vi "chamber control mockup.vi"() -> ()   [LabVIEW 2013]
uses:
  dconners svn copy/TemperatureLogger/controls/TabControl.ctl
  dconners svn copy/TemperatureLogger/controls/TemperatureControlCluster2.ctl
  dconners svn copy/TemperatureLogger/controls/outputcluster.ctl
panel:
  in  "Save freq (seconds between samples)":dbl
  in  "Log note":bool
  in  "Notes":string
  out "Chiller alarm":bool
  out "Free GB":dbl
  in  "Data storage location":path
  in  "Chiller flow speed":u16(ring) items=["Low", "Medium", "High"]
  in  "Chiller process value":dbl
  in  "Chiller setpoint":dbl
  out "Profile running":bool
  in  "Big Chamber setpoint 3":dbl
  out "Big Chamber process value 3":dbl
  in  "Little Chamber setpoint 3":dbl
  out "Little Chamber process value 3":dbl
  in  "Big Chamber setpoint 2":dbl
  out "Big Chamber process value 2":dbl
  in  "Little Chamber setpoint 2":dbl
  out "Little Chamber process value 2":dbl
  in  "Relay 3":bool
  in  "Relay 2":bool
  in  "Relay 4":bool
  in  "Relay 1":bool
  in  "Tab Control":T1(tab)
  in  "Popout to new window 6":bool
  in  "Tab Control 7":T2
  in  "String 18":string
  in  "String 17":string
  in  "String 16":string
  in  "String 15":string
  in  "String 14":string
  in  "String 13":string
  in  "String 12":string
  in  "String 11":string
  in  "String 10":string
  in  "String 9":string
  in  "String 8":string
  in  "String 7":string
  in  "String 6":string
  in  "String 5":string
  in  "String 4":string
  in  "String 3":string
  in  "String 2":string
  out "DisplayCluster 6":T3={"Thermometer 2"=0.0, "Temperature Chart 4"=[{"t0"=timestamp(3419368924.4957023 s since 1904-01-01), "dt"=1.0, "Y"=[23.012484100583272], "attributes"=variant("NI_ChannelName"=variant(string "ai0"), "NI_UnitDescription"=variant(string "Deg C"))}, {"t0"=timestamp(3419368924.4957023 s since 1904-01-01), "dt"=1.0, "Y"=[23.20749068697193], "attributes"=variant("NI_ChannelName"=variant(string "ai1"), "NI_UnitDescription"=variant(string "Deg C"))}, {"t0"=timestamp(3419368924.4957023 s since 1904-01-01), "dt"=1.0, "Y"=[23.4994745351067], "attributes"=variant("NI_ChannelName"=variant(string "ai2"), "NI_UnitDescription"=variant(string "Deg C"))}], "Alarm"=FALSE, "Thermometer"=0.0, "File Path"=""} {"Thermometer" scale=0.0..100.0; "Thermometer 2" scale=0.0..100.0}
  out "Temperatures 6":dbl[](array[numeric]) format="%#.2f"
  in  "Save Data 6":bool=TRUE
  in  "Log File Path 6":path=path "c:/Temp/Data"
  out "DAQmx Device Name 6":tag="cDAQ2Mod1"
  out "Errors 6":errorcluster
  in  "Number of channels 6":i32=1 min=1 max=16 step=1
  in  "sample/S 6":dbl=1.0 min=0.1 max=75.0 step=0.1
  in  "Alarm recipients 6":string[](array[string])=["dconnors@intven.com"]
  in  "Upper Alarm 6":dbl=150.0
  in  "Lower Alarm 6":dbl=-150.0
  in  "Email Enable 6":bool
  in  "Cluster 7":T4={"Channel Setup"=[{"Channel #"=1, "TC TYPE"=10086, "Name"=""}, {"Channel #"=5, "TC TYPE"=10086, "Name"=""}, {"Channel #"=9, "TC TYPE"=10086, "Name"=""}, {"Channel #"=13, "TC TYPE"=10086, "Name"=""}], "Channel Setup 2"=[{"Channel #"=1, "TC TYPE"=10086, "Name"=""}, {"Channel #"=5, "TC TYPE"=10086, "Name"=""}, {"Channel #"=9, "TC TYPE"=10086, "Name"=""}, {"Channel #"=13, "TC TYPE"=10086, "Name"=""}], "Channel Setup 3"=[{"Channel #"=1, "TC TYPE"=10086, "Name"=""}, {"Channel #"=5, "TC TYPE"=10086, "Name"=""}, {"Channel #"=9, "TC TYPE"=10086, "Name"=""}, {"Channel #"=13, "TC TYPE"=10086, "Name"=""}], "Channel Setup 4"=[{"Channel #"=1, "TC TYPE"=10086, "Name"=""}, {"Channel #"=5, "TC TYPE"=10086, "Name"=""}, {"Channel #"=9, "TC TYPE"=10086, "Name"=""}, {"Channel #"=13, "TC TYPE"=10086, "Name"=""}]} {"Channel Setup 4"."TC TYPE" items=["J"=10072, "K"=10073, "N"=10077, "R"=10082, "S"=10085, "T"=10086, "B"=10047, "E"=10055]; "Channel Setup 4"."Channel #" min=1 max=16 step=1; "Channel Setup 3"."TC TYPE" items=["J"=10072, "K"=10073, "N"=10077, "R"=10082, "S"=10085, "T"=10086, "B"=10047, "E"=10055]; "Channel Setup 3"."Channel #" min=1 max=16 step=1; "Channel Setup 2"."TC TYPE" items=["J"=10072, "K"=10073, "N"=10077, "R"=10082, "S"=10085, "T"=10086, "B"=10047, "E"=10055]; "Channel Setup 2"."Channel #" min=1 max=16 step=1; "Channel Setup"."TC TYPE" items=["J"=10072, "K"=10073, "N"=10077, "R"=10082, "S"=10085, "T"=10086, "B"=10047, "E"=10055]; "Channel Setup"."Channel #" min=1 max=16 step=1}
  out "IP Address 6":string=" "
  in  "Minutes between emails 6":dbl=10.0
  in  "Popout to new window":bool
  in  "Tab Control 2":T2
  in  "String":string
  out "DisplayCluster":T3={"Thermometer 2"=0.0, "Temperature Chart 4"=[{"t0"=timestamp(3419368924.4957023 s since 1904-01-01), "dt"=1.0, "Y"=[23.012484100583272], "attributes"=variant("NI_ChannelName"=variant(string "ai0"), "NI_UnitDescription"=variant(string "Deg C"))}, {"t0"=timestamp(3419368924.4957023 s since 1904-01-01), "dt"=1.0, "Y"=[23.20749068697193], "attributes"=variant("NI_ChannelName"=variant(string "ai1"), "NI_UnitDescription"=variant(string "Deg C"))}, {"t0"=timestamp(3419368924.4957023 s since 1904-01-01), "dt"=1.0, "Y"=[23.4994745351067], "attributes"=variant("NI_ChannelName"=variant(string "ai2"), "NI_UnitDescription"=variant(string "Deg C"))}], "Alarm"=FALSE, "Thermometer"=0.0, "File Path"=""} {"Thermometer" scale=0.0..100.0; "Thermometer 2" scale=0.0..100.0}
  out "Temperatures":dbl[](array[numeric]) format="%#.2f"
  in  "Reset max/min":bool
  in  "Save Data":bool=TRUE
  in  "Log File Path":path=path "c:/Temp/Data"
  out "DAQmx Device Name":tag="cDAQ2Mod1"
  out "Errors":errorcluster
  in  "Number of channels":i32=1 min=1 max=16 step=1
  in  "sample/S":dbl=1.0 min=0.1 max=75.0 step=0.1
  in  "Alarm recipients":string[](array[string])=["dconnors@intven.com"]
  in  "Upper Alarm":dbl=150.0
  in  "Lower Alarm":dbl=-150.0
  in  "Email Enable":bool
  in  "Cluster 2":T4={"Channel Setup"=[{"Channel #"=1, "TC TYPE"=10086, "Name"=""}, {"Channel #"=5, "TC TYPE"=10086, "Name"=""}, {"Channel #"=9, "TC TYPE"=10086, "Name"=""}, {"Channel #"=13, "TC TYPE"=10086, "Name"=""}], "Channel Setup 2"=[{"Channel #"=1, "TC TYPE"=10086, "Name"=""}, {"Channel #"=5, "TC TYPE"=10086, "Name"=""}, {"Channel #"=9, "TC TYPE"=10086, "Name"=""}, {"Channel #"=13, "TC TYPE"=10086, "Name"=""}], "Channel Setup 3"=[{"Channel #"=1, "TC TYPE"=10086, "Name"=""}, {"Channel #"=5, "TC TYPE"=10086, "Name"=""}, {"Channel #"=9, "TC TYPE"=10086, "Name"=""}, {"Channel #"=13, "TC TYPE"=10086, "Name"=""}], "Channel Setup 4"=[{"Channel #"=1, "TC TYPE"=10086, "Name"=""}, {"Channel #"=5, "TC TYPE"=10086, "Name"=""}, {"Channel #"=9, "TC TYPE"=10086, "Name"=""}, {"Channel #"=13, "TC TYPE"=10086, "Name"=""}]} {"Channel Setup 4"."TC TYPE" items=["J"=10072, "K"=10073, "N"=10077, "R"=10082, "S"=10085, "T"=10086, "B"=10047, "E"=10055]; "Channel Setup 4"."Channel #" min=1 max=16 step=1; "Channel Setup 3"."TC TYPE" items=["J"=10072, "K"=10073, "N"=10077, "R"=10082, "S"=10085, "T"=10086, "B"=10047, "E"=10055]; "Channel Setup 3"."Channel #" min=1 max=16 step=1; "Channel Setup 2"."TC TYPE" items=["J"=10072, "K"=10073, "N"=10077, "R"=10082, "S"=10085, "T"=10086, "B"=10047, "E"=10055]; "Channel Setup 2"."Channel #" min=1 max=16 step=1; "Channel Setup"."TC TYPE" items=["J"=10072, "K"=10073, "N"=10077, "R"=10082, "S"=10085, "T"=10086, "B"=10047, "E"=10055]; "Channel Setup"."Channel #" min=1 max=16 step=1}
  out "IP Address":string=" "
  in  "Minutes between emails":dbl=10.0
  in  "Popout to new window 7":bool
  in  "Tab Control 8":T2
  in  "String 36":string
  in  "String 35":string
  in  "String 34":string
  in  "String 33":string
  in  "String 32":string
  in  "String 31":string
  in  "String 30":string
  in  "String 29":string
  in  "String 28":string
  in  "String 27":string
  in  "String 26":string
  in  "String 25":string
  in  "String 24":string
  in  "String 23":string
  in  "String 22":string
  in  "String 21":string
  in  "String 20":string
  out "DisplayCluster 7":T3={"Thermometer 2"=0.0, "Temperature Chart 4"=[{"t0"=timestamp(3419368924.4957023 s since 1904-01-01), "dt"=1.0, "Y"=[23.012484100583272], "attributes"=variant("NI_ChannelName"=variant(string "ai0"), "NI_UnitDescription"=variant(string "Deg C"))}, {"t0"=timestamp(3419368924.4957023 s since 1904-01-01), "dt"=1.0, "Y"=[23.20749068697193], "attributes"=variant("NI_ChannelName"=variant(string "ai1"), "NI_UnitDescription"=variant(string "Deg C"))}, {"t0"=timestamp(3419368924.4957023 s since 1904-01-01), "dt"=1.0, "Y"=[23.4994745351067], "attributes"=variant("NI_ChannelName"=variant(string "ai2"), "NI_UnitDescription"=variant(string "Deg C"))}], "Alarm"=FALSE, "Thermometer"=0.0, "File Path"=""} {"Thermometer" scale=0.0..100.0; "Thermometer 2" scale=0.0..100.0}
  out "Temperatures 7":dbl[](array[numeric]) format="%#.2f"
  in  "Save Data 7":bool=TRUE
  in  "Log File Path 7":path=path "c:/Temp/Data"
  out "DAQmx Device Name 7":tag="cDAQ2Mod1"
  out "Errors 7":errorcluster
  in  "Number of channels 7":i32=1 min=1 max=16 step=1
  in  "sample/S 7":dbl=1.0 min=0.1 max=75.0 step=0.1
  in  "Alarm recipients 7":string[](array[string])=["dconnors@intven.com"]
  in  "Upper Alarm 7":dbl=150.0
  in  "Lower Alarm 7":dbl=-150.0
  in  "Email Enable 7":bool
  in  "Cluster 8":T4={"Channel Setup"=[{"Channel #"=1, "TC TYPE"=10086, "Name"=""}, {"Channel #"=5, "TC TYPE"=10086, "Name"=""}, {"Channel #"=9, "TC TYPE"=10086, "Name"=""}, {"Channel #"=13, "TC TYPE"=10086, "Name"=""}], "Channel Setup 2"=[{"Channel #"=1, "TC TYPE"=10086, "Name"=""}, {"Channel #"=5, "TC TYPE"=10086, "Name"=""}, {"Channel #"=9, "TC TYPE"=10086, "Name"=""}, {"Channel #"=13, "TC TYPE"=10086, "Name"=""}], "Channel Setup 3"=[{"Channel #"=1, "TC TYPE"=10086, "Name"=""}, {"Channel #"=5, "TC TYPE"=10086, "Name"=""}, {"Channel #"=9, "TC TYPE"=10086, "Name"=""}, {"Channel #"=13, "TC TYPE"=10086, "Name"=""}], "Channel Setup 4"=[{"Channel #"=1, "TC TYPE"=10086, "Name"=""}, {"Channel #"=5, "TC TYPE"=10086, "Name"=""}, {"Channel #"=9, "TC TYPE"=10086, "Name"=""}, {"Channel #"=13, "TC TYPE"=10086, "Name"=""}]} {"Channel Setup 4"."TC TYPE" items=["J"=10072, "K"=10073, "N"=10077, "R"=10082, "S"=10085, "T"=10086, "B"=10047, "E"=10055]; "Channel Setup 4"."Channel #" min=1 max=16 step=1; "Channel Setup 3"."TC TYPE" items=["J"=10072, "K"=10073, "N"=10077, "R"=10082, "S"=10085, "T"=10086, "B"=10047, "E"=10055]; "Channel Setup 3"."Channel #" min=1 max=16 step=1; "Channel Setup 2"."TC TYPE" items=["J"=10072, "K"=10073, "N"=10077, "R"=10082, "S"=10085, "T"=10086, "B"=10047, "E"=10055]; "Channel Setup 2"."Channel #" min=1 max=16 step=1; "Channel Setup"."TC TYPE" items=["J"=10072, "K"=10073, "N"=10077, "R"=10082, "S"=10085, "T"=10086, "B"=10047, "E"=10055]; "Channel Setup"."Channel #" min=1 max=16 step=1}
  out "IP Address 7":string=" "
  in  "Minutes between emails 7":dbl=10.0
  in  "Popout to new window 2":bool
  in  "Tab Control 3":T2
  in  "String 19":string
  out "DisplayCluster 2":T3={"Thermometer 2"=0.0, "Temperature Chart 4"=[{"t0"=timestamp(3419368924.4957023 s since 1904-01-01), "dt"=1.0, "Y"=[23.012484100583272], "attributes"=variant("NI_ChannelName"=variant(string "ai0"), "NI_UnitDescription"=variant(string "Deg C"))}, {"t0"=timestamp(3419368924.4957023 s since 1904-01-01), "dt"=1.0, "Y"=[23.20749068697193], "attributes"=variant("NI_ChannelName"=variant(string "ai1"), "NI_UnitDescription"=variant(string "Deg C"))}, {"t0"=timestamp(3419368924.4957023 s since 1904-01-01), "dt"=1.0, "Y"=[23.4994745351067], "attributes"=variant("NI_ChannelName"=variant(string "ai2"), "NI_UnitDescription"=variant(string "Deg C"))}], "Alarm"=FALSE, "Thermometer"=0.0, "File Path"=""} {"Thermometer" scale=0.0..100.0; "Thermometer 2" scale=0.0..100.0}
  out "Temperatures 2":dbl[](array[numeric]) format="%#.2f"
  in  "Reset max/min 2":bool
  in  "Save Data 2":bool=TRUE
  in  "Log File Path 2":path=path "c:/Temp/Data"
  out "DAQmx Device Name 2":tag="cDAQ2Mod1"
  out "Errors 2":errorcluster
  in  "Number of channels 2":i32=1 min=1 max=16 step=1
  in  "sample/S 2":dbl=1.0 min=0.1 max=75.0 step=0.1
  in  "Alarm recipients 2":string[](array[string])=["dconnors@intven.com"]
  in  "Upper Alarm 2":dbl=150.0
  in  "Lower Alarm 2":dbl=-150.0
  in  "Email Enable 2":bool
  in  "Cluster 3":T4={"Channel Setup"=[{"Channel #"=1, "TC TYPE"=10086, "Name"=""}, {"Channel #"=5, "TC TYPE"=10086, "Name"=""}, {"Channel #"=9, "TC TYPE"=10086, "Name"=""}, {"Channel #"=13, "TC TYPE"=10086, "Name"=""}], "Channel Setup 2"=[{"Channel #"=1, "TC TYPE"=10086, "Name"=""}, {"Channel #"=5, "TC TYPE"=10086, "Name"=""}, {"Channel #"=9, "TC TYPE"=10086, "Name"=""}, {"Channel #"=13, "TC TYPE"=10086, "Name"=""}], "Channel Setup 3"=[{"Channel #"=1, "TC TYPE"=10086, "Name"=""}, {"Channel #"=5, "TC TYPE"=10086, "Name"=""}, {"Channel #"=9, "TC TYPE"=10086, "Name"=""}, {"Channel #"=13, "TC TYPE"=10086, "Name"=""}], "Channel Setup 4"=[{"Channel #"=1, "TC TYPE"=10086, "Name"=""}, {"Channel #"=5, "TC TYPE"=10086, "Name"=""}, {"Channel #"=9, "TC TYPE"=10086, "Name"=""}, {"Channel #"=13, "TC TYPE"=10086, "Name"=""}]} {"Channel Setup 4"."TC TYPE" items=["J"=10072, "K"=10073, "N"=10077, "R"=10082, "S"=10085, "T"=10086, "B"=10047, "E"=10055]; "Channel Setup 4"."Channel #" min=1 max=16 step=1; "Channel Setup 3"."TC TYPE" items=["J"=10072, "K"=10073, "N"=10077, "R"=10082, "S"=10085, "T"=10086, "B"=10047, "E"=10055]; "Channel Setup 3"."Channel #" min=1 max=16 step=1; "Channel Setup 2"."TC TYPE" items=["J"=10072, "K"=10073, "N"=10077, "R"=10082, "S"=10085, "T"=10086, "B"=10047, "E"=10055]; "Channel Setup 2"."Channel #" min=1 max=16 step=1; "Channel Setup"."TC TYPE" items=["J"=10072, "K"=10073, "N"=10077, "R"=10082, "S"=10085, "T"=10086, "B"=10047, "E"=10055]; "Channel Setup"."Channel #" min=1 max=16 step=1}
  out "IP Address 2":string=" "
  in  "Minutes between emails 2":dbl=10.0
  in  "Popout to new window 8":bool
  in  "Tab Control 9":T2
  in  "String 54":string
  in  "String 53":string
  in  "String 52":string
  in  "String 51":string
  in  "String 50":string
  in  "String 49":string
  in  "String 48":string
  in  "String 47":string
  in  "String 46":string
  in  "String 45":string
  in  "String 44":string
  in  "String 43":string
  in  "String 42":string
  in  "String 41":string
  in  "String 40":string
  in  "String 39":string
  in  "String 38":string
  out "DisplayCluster 8":T3={"Thermometer 2"=0.0, "Temperature Chart 4"=[{"t0"=timestamp(3419368924.4957023 s since 1904-01-01), "dt"=1.0, "Y"=[23.012484100583272], "attributes"=variant("NI_ChannelName"=variant(string "ai0"), "NI_UnitDescription"=variant(string "Deg C"))}, {"t0"=timestamp(3419368924.4957023 s since 1904-01-01), "dt"=1.0, "Y"=[23.20749068697193], "attributes"=variant("NI_ChannelName"=variant(string "ai1"), "NI_UnitDescription"=variant(string "Deg C"))}, {"t0"=timestamp(3419368924.4957023 s since 1904-01-01), "dt"=1.0, "Y"=[23.4994745351067], "attributes"=variant("NI_ChannelName"=variant(string "ai2"), "NI_UnitDescription"=variant(string "Deg C"))}], "Alarm"=FALSE, "Thermometer"=0.0, "File Path"=""} {"Thermometer" scale=0.0..100.0; "Thermometer 2" scale=0.0..100.0}
  out "Temperatures 8":dbl[](array[numeric]) format="%#.2f"
  in  "Save Data 8":bool=TRUE
  in  "Log File Path 8":path=path "c:/Temp/Data"
  out "DAQmx Device Name 8":tag="cDAQ2Mod1"
  out "Errors 8":errorcluster
  in  "Number of channels 8":i32=1 min=1 max=16 step=1
  in  "sample/S 8":dbl=1.0 min=0.1 max=75.0 step=0.1
  in  "Alarm recipients 8":string[](array[string])=["dconnors@intven.com"]
  in  "Upper Alarm 8":dbl=150.0
  in  "Lower Alarm 8":dbl=-150.0
  in  "Email Enable 8":bool
  in  "Cluster 9":T4={"Channel Setup"=[{"Channel #"=1, "TC TYPE"=10086, "Name"=""}, {"Channel #"=5, "TC TYPE"=10086, "Name"=""}, {"Channel #"=9, "TC TYPE"=10086, "Name"=""}, {"Channel #"=13, "TC TYPE"=10086, "Name"=""}], "Channel Setup 2"=[{"Channel #"=1, "TC TYPE"=10086, "Name"=""}, {"Channel #"=5, "TC TYPE"=10086, "Name"=""}, {"Channel #"=9, "TC TYPE"=10086, "Name"=""}, {"Channel #"=13, "TC TYPE"=10086, "Name"=""}], "Channel Setup 3"=[{"Channel #"=1, "TC TYPE"=10086, "Name"=""}, {"Channel #"=5, "TC TYPE"=10086, "Name"=""}, {"Channel #"=9, "TC TYPE"=10086, "Name"=""}, {"Channel #"=13, "TC TYPE"=10086, "Name"=""}], "Channel Setup 4"=[{"Channel #"=1, "TC TYPE"=10086, "Name"=""}, {"Channel #"=5, "TC TYPE"=10086, "Name"=""}, {"Channel #"=9, "TC TYPE"=10086, "Name"=""}, {"Channel #"=13, "TC TYPE"=10086, "Name"=""}]} {"Channel Setup 4"."TC TYPE" items=["J"=10072, "K"=10073, "N"=10077, "R"=10082, "S"=10085, "T"=10086, "B"=10047, "E"=10055]; "Channel Setup 4"."Channel #" min=1 max=16 step=1; "Channel Setup 3"."TC TYPE" items=["J"=10072, "K"=10073, "N"=10077, "R"=10082, "S"=10085, "T"=10086, "B"=10047, "E"=10055]; "Channel Setup 3"."Channel #" min=1 max=16 step=1; "Channel Setup 2"."TC TYPE" items=["J"=10072, "K"=10073, "N"=10077, "R"=10082, "S"=10085, "T"=10086, "B"=10047, "E"=10055]; "Channel Setup 2"."Channel #" min=1 max=16 step=1; "Channel Setup"."TC TYPE" items=["J"=10072, "K"=10073, "N"=10077, "R"=10082, "S"=10085, "T"=10086, "B"=10047, "E"=10055]; "Channel Setup"."Channel #" min=1 max=16 step=1}
  out "IP Address 8":string=" "
  in  "Minutes between emails 8":dbl=10.0
  in  "Popout to new window 3":bool
  in  "Tab Control 4":T2
  in  "String 37":string
  out "DisplayCluster 3":T3={"Thermometer 2"=0.0, "Temperature Chart 4"=[{"t0"=timestamp(3419368924.4957023 s since 1904-01-01), "dt"=1.0, "Y"=[23.012484100583272], "attributes"=variant("NI_ChannelName"=variant(string "ai0"), "NI_UnitDescription"=variant(string "Deg C"))}, {"t0"=timestamp(3419368924.4957023 s since 1904-01-01), "dt"=1.0, "Y"=[23.20749068697193], "attributes"=variant("NI_ChannelName"=variant(string "ai1"), "NI_UnitDescription"=variant(string "Deg C"))}, {"t0"=timestamp(3419368924.4957023 s since 1904-01-01), "dt"=1.0, "Y"=[23.4994745351067], "attributes"=variant("NI_ChannelName"=variant(string "ai2"), "NI_UnitDescription"=variant(string "Deg C"))}], "Alarm"=FALSE, "Thermometer"=0.0, "File Path"=""} {"Thermometer" scale=0.0..100.0; "Thermometer 2" scale=0.0..100.0}
  out "Temperatures 3":dbl[](array[numeric]) format="%#.2f"
  in  "Reset max/min 3":bool
  in  "Save Data 3":bool=TRUE
  in  "Log File Path 3":path=path "c:/Temp/Data"
  out "DAQmx Device Name 3":tag="cDAQ2Mod1"
  out "Errors 3":errorcluster
  in  "Number of channels 3":i32=1 min=1 max=16 step=1
  in  "sample/S 3":dbl=1.0 min=0.1 max=75.0 step=0.1
  in  "Alarm recipients 3":string[](array[string])=["dconnors@intven.com"]
  in  "Upper Alarm 3":dbl=150.0
  in  "Lower Alarm 3":dbl=-150.0
  in  "Email Enable 3":bool
  in  "Cluster 4":T4={"Channel Setup"=[{"Channel #"=1, "TC TYPE"=10086, "Name"=""}, {"Channel #"=5, "TC TYPE"=10086, "Name"=""}, {"Channel #"=9, "TC TYPE"=10086, "Name"=""}, {"Channel #"=13, "TC TYPE"=10086, "Name"=""}], "Channel Setup 2"=[{"Channel #"=1, "TC TYPE"=10086, "Name"=""}, {"Channel #"=5, "TC TYPE"=10086, "Name"=""}, {"Channel #"=9, "TC TYPE"=10086, "Name"=""}, {"Channel #"=13, "TC TYPE"=10086, "Name"=""}], "Channel Setup 3"=[{"Channel #"=1, "TC TYPE"=10086, "Name"=""}, {"Channel #"=5, "TC TYPE"=10086, "Name"=""}, {"Channel #"=9, "TC TYPE"=10086, "Name"=""}, {"Channel #"=13, "TC TYPE"=10086, "Name"=""}], "Channel Setup 4"=[{"Channel #"=1, "TC TYPE"=10086, "Name"=""}, {"Channel #"=5, "TC TYPE"=10086, "Name"=""}, {"Channel #"=9, "TC TYPE"=10086, "Name"=""}, {"Channel #"=13, "TC TYPE"=10086, "Name"=""}]} {"Channel Setup 4"."TC TYPE" items=["J"=10072, "K"=10073, "N"=10077, "R"=10082, "S"=10085, "T"=10086, "B"=10047, "E"=10055]; "Channel Setup 4"."Channel #" min=1 max=16 step=1; "Channel Setup 3"."TC TYPE" items=["J"=10072, "K"=10073, "N"=10077, "R"=10082, "S"=10085, "T"=10086, "B"=10047, "E"=10055]; "Channel Setup 3"."Channel #" min=1 max=16 step=1; "Channel Setup 2"."TC TYPE" items=["J"=10072, "K"=10073, "N"=10077, "R"=10082, "S"=10085, "T"=10086, "B"=10047, "E"=10055]; "Channel Setup 2"."Channel #" min=1 max=16 step=1; "Channel Setup"."TC TYPE" items=["J"=10072, "K"=10073, "N"=10077, "R"=10082, "S"=10085, "T"=10086, "B"=10047, "E"=10055]; "Channel Setup"."Channel #" min=1 max=16 step=1}
  out "IP Address 3":string=" "
  in  "Minutes between emails 3":dbl=10.0
  in  "Popout to new window 9":bool
  in  "Tab Control 10":T2
  in  "String 72":string
  in  "String 71":string
  in  "String 70":string
  in  "String 69":string
  in  "String 68":string
  in  "String 67":string
  in  "String 66":string
  in  "String 65":string
  in  "String 64":string
  in  "String 63":string
  in  "String 62":string
  in  "String 61":string
  in  "String 60":string
  in  "String 59":string
  in  "String 58":string
  in  "String 57":string
  in  "String 56":string
  out "DisplayCluster 9":T3={"Thermometer 2"=0.0, "Temperature Chart 4"=[{"t0"=timestamp(3419368924.4957023 s since 1904-01-01), "dt"=1.0, "Y"=[23.012484100583272], "attributes"=variant("NI_ChannelName"=variant(string "ai0"), "NI_UnitDescription"=variant(string "Deg C"))}, {"t0"=timestamp(3419368924.4957023 s since 1904-01-01), "dt"=1.0, "Y"=[23.20749068697193], "attributes"=variant("NI_ChannelName"=variant(string "ai1"), "NI_UnitDescription"=variant(string "Deg C"))}, {"t0"=timestamp(3419368924.4957023 s since 1904-01-01), "dt"=1.0, "Y"=[23.4994745351067], "attributes"=variant("NI_ChannelName"=variant(string "ai2"), "NI_UnitDescription"=variant(string "Deg C"))}], "Alarm"=FALSE, "Thermometer"=0.0, "File Path"=""} {"Thermometer" scale=0.0..100.0; "Thermometer 2" scale=0.0..100.0}
  out "Temperatures 9":dbl[](array[numeric]) format="%#.2f"
  in  "Save Data 9":bool=TRUE
  in  "Log File Path 9":path=path "c:/Temp/Data"
  out "DAQmx Device Name 9":tag="cDAQ2Mod1"
  out "Errors 9":errorcluster
  in  "Number of channels 9":i32=1 min=1 max=16 step=1
  in  "sample/S 9":dbl=1.0 min=0.1 max=75.0 step=0.1
  in  "Alarm recipients 9":string[](array[string])=["dconnors@intven.com"]
  in  "Upper Alarm 9":dbl=150.0
  in  "Lower Alarm 9":dbl=-150.0
  in  "Email Enable 9":bool
  in  "Cluster 10":T4={"Channel Setup"=[{"Channel #"=1, "TC TYPE"=10086, "Name"=""}, {"Channel #"=5, "TC TYPE"=10086, "Name"=""}, {"Channel #"=9, "TC TYPE"=10086, "Name"=""}, {"Channel #"=13, "TC TYPE"=10086, "Name"=""}], "Channel Setup 2"=[{"Channel #"=1, "TC TYPE"=10086, "Name"=""}, {"Channel #"=5, "TC TYPE"=10086, "Name"=""}, {"Channel #"=9, "TC TYPE"=10086, "Name"=""}, {"Channel #"=13, "TC TYPE"=10086, "Name"=""}], "Channel Setup 3"=[{"Channel #"=1, "TC TYPE"=10086, "Name"=""}, {"Channel #"=5, "TC TYPE"=10086, "Name"=""}, {"Channel #"=9, "TC TYPE"=10086, "Name"=""}, {"Channel #"=13, "TC TYPE"=10086, "Name"=""}], "Channel Setup 4"=[{"Channel #"=1, "TC TYPE"=10086, "Name"=""}, {"Channel #"=5, "TC TYPE"=10086, "Name"=""}, {"Channel #"=9, "TC TYPE"=10086, "Name"=""}, {"Channel #"=13, "TC TYPE"=10086, "Name"=""}]} {"Channel Setup 4"."TC TYPE" items=["J"=10072, "K"=10073, "N"=10077, "R"=10082, "S"=10085, "T"=10086, "B"=10047, "E"=10055]; "Channel Setup 4"."Channel #" min=1 max=16 step=1; "Channel Setup 3"."TC TYPE" items=["J"=10072, "K"=10073, "N"=10077, "R"=10082, "S"=10085, "T"=10086, "B"=10047, "E"=10055]; "Channel Setup 3"."Channel #" min=1 max=16 step=1; "Channel Setup 2"."TC TYPE" items=["J"=10072, "K"=10073, "N"=10077, "R"=10082, "S"=10085, "T"=10086, "B"=10047, "E"=10055]; "Channel Setup 2"."Channel #" min=1 max=16 step=1; "Channel Setup"."TC TYPE" items=["J"=10072, "K"=10073, "N"=10077, "R"=10082, "S"=10085, "T"=10086, "B"=10047, "E"=10055]; "Channel Setup"."Channel #" min=1 max=16 step=1}
  out "IP Address 9":string=" "
  in  "Minutes between emails 9":dbl=10.0
  in  "Popout to new window 4":bool
  in  "Tab Control 5":T2
  in  "String 55":string
  out "DisplayCluster 4":T3={"Thermometer 2"=0.0, "Temperature Chart 4"=[{"t0"=timestamp(3419368924.4957023 s since 1904-01-01), "dt"=1.0, "Y"=[23.012484100583272], "attributes"=variant("NI_ChannelName"=variant(string "ai0"), "NI_UnitDescription"=variant(string "Deg C"))}, {"t0"=timestamp(3419368924.4957023 s since 1904-01-01), "dt"=1.0, "Y"=[23.20749068697193], "attributes"=variant("NI_ChannelName"=variant(string "ai1"), "NI_UnitDescription"=variant(string "Deg C"))}, {"t0"=timestamp(3419368924.4957023 s since 1904-01-01), "dt"=1.0, "Y"=[23.4994745351067], "attributes"=variant("NI_ChannelName"=variant(string "ai2"), "NI_UnitDescription"=variant(string "Deg C"))}], "Alarm"=FALSE, "Thermometer"=0.0, "File Path"=""} {"Thermometer" scale=0.0..100.0; "Thermometer 2" scale=0.0..100.0}
  out "Temperatures 4":dbl[](array[numeric]) format="%#.2f"
  in  "Reset max/min 4":bool
  in  "Save Data 4":bool=TRUE
  in  "Log File Path 4":path=path "c:/Temp/Data"
  out "DAQmx Device Name 4":tag="cDAQ2Mod1"
  out "Errors 4":errorcluster
  in  "Number of channels 4":i32=1 min=1 max=16 step=1
  in  "sample/S 4":dbl=1.0 min=0.1 max=75.0 step=0.1
  in  "Alarm recipients 4":string[](array[string])=["dconnors@intven.com"]
  in  "Upper Alarm 4":dbl=150.0
  in  "Lower Alarm 4":dbl=-150.0
  in  "Email Enable 4":bool
  in  "Cluster 5":T4={"Channel Setup"=[{"Channel #"=1, "TC TYPE"=10086, "Name"=""}, {"Channel #"=5, "TC TYPE"=10086, "Name"=""}, {"Channel #"=9, "TC TYPE"=10086, "Name"=""}, {"Channel #"=13, "TC TYPE"=10086, "Name"=""}], "Channel Setup 2"=[{"Channel #"=1, "TC TYPE"=10086, "Name"=""}, {"Channel #"=5, "TC TYPE"=10086, "Name"=""}, {"Channel #"=9, "TC TYPE"=10086, "Name"=""}, {"Channel #"=13, "TC TYPE"=10086, "Name"=""}], "Channel Setup 3"=[{"Channel #"=1, "TC TYPE"=10086, "Name"=""}, {"Channel #"=5, "TC TYPE"=10086, "Name"=""}, {"Channel #"=9, "TC TYPE"=10086, "Name"=""}, {"Channel #"=13, "TC TYPE"=10086, "Name"=""}], "Channel Setup 4"=[{"Channel #"=1, "TC TYPE"=10086, "Name"=""}, {"Channel #"=5, "TC TYPE"=10086, "Name"=""}, {"Channel #"=9, "TC TYPE"=10086, "Name"=""}, {"Channel #"=13, "TC TYPE"=10086, "Name"=""}]} {"Channel Setup 4"."TC TYPE" items=["J"=10072, "K"=10073, "N"=10077, "R"=10082, "S"=10085, "T"=10086, "B"=10047, "E"=10055]; "Channel Setup 4"."Channel #" min=1 max=16 step=1; "Channel Setup 3"."TC TYPE" items=["J"=10072, "K"=10073, "N"=10077, "R"=10082, "S"=10085, "T"=10086, "B"=10047, "E"=10055]; "Channel Setup 3"."Channel #" min=1 max=16 step=1; "Channel Setup 2"."TC TYPE" items=["J"=10072, "K"=10073, "N"=10077, "R"=10082, "S"=10085, "T"=10086, "B"=10047, "E"=10055]; "Channel Setup 2"."Channel #" min=1 max=16 step=1; "Channel Setup"."TC TYPE" items=["J"=10072, "K"=10073, "N"=10077, "R"=10082, "S"=10085, "T"=10086, "B"=10047, "E"=10055]; "Channel Setup"."Channel #" min=1 max=16 step=1}
  out "IP Address 4":string=" "
  in  "Minutes between emails 4":dbl=10.0
  in  "Popout to new window 10":bool
  in  "Tab Control 11":T2
  in  "String 90":string
  in  "String 89":string
  in  "String 88":string
  in  "String 87":string
  in  "String 86":string
  in  "String 85":string
  in  "String 84":string
  in  "String 83":string
  in  "String 82":string
  in  "String 81":string
  in  "String 80":string
  in  "String 79":string
  in  "String 78":string
  in  "String 77":string
  in  "String 76":string
  in  "String 75":string
  in  "String 74":string
  out "DisplayCluster 10":T3={"Thermometer 2"=0.0, "Temperature Chart 4"=[{"t0"=timestamp(3419368924.4957023 s since 1904-01-01), "dt"=1.0, "Y"=[23.012484100583272], "attributes"=variant("NI_ChannelName"=variant(string "ai0"), "NI_UnitDescription"=variant(string "Deg C"))}, {"t0"=timestamp(3419368924.4957023 s since 1904-01-01), "dt"=1.0, "Y"=[23.20749068697193], "attributes"=variant("NI_ChannelName"=variant(string "ai1"), "NI_UnitDescription"=variant(string "Deg C"))}, {"t0"=timestamp(3419368924.4957023 s since 1904-01-01), "dt"=1.0, "Y"=[23.4994745351067], "attributes"=variant("NI_ChannelName"=variant(string "ai2"), "NI_UnitDescription"=variant(string "Deg C"))}], "Alarm"=FALSE, "Thermometer"=0.0, "File Path"=""} {"Thermometer" scale=0.0..100.0; "Thermometer 2" scale=0.0..100.0}
  out "Temperatures 10":dbl[](array[numeric]) format="%#.2f"
  in  "Save Data 10":bool=TRUE
  in  "Log File Path 10":path=path "c:/Temp/Data"
  out "DAQmx Device Name 10":tag="cDAQ2Mod1"
  out "Errors 10":errorcluster
  in  "Number of channels 10":i32=1 min=1 max=16 step=1
  in  "sample/S 10":dbl=1.0 min=0.1 max=75.0 step=0.1
  in  "Alarm recipients 10":string[](array[string])=["dconnors@intven.com"]
  in  "Upper Alarm 10":dbl=150.0
  in  "Lower Alarm 10":dbl=-150.0
  in  "Email Enable 10":bool
  in  "Cluster 11":T4={"Channel Setup"=[{"Channel #"=1, "TC TYPE"=10086, "Name"=""}, {"Channel #"=5, "TC TYPE"=10086, "Name"=""}, {"Channel #"=9, "TC TYPE"=10086, "Name"=""}, {"Channel #"=13, "TC TYPE"=10086, "Name"=""}], "Channel Setup 2"=[{"Channel #"=1, "TC TYPE"=10086, "Name"=""}, {"Channel #"=5, "TC TYPE"=10086, "Name"=""}, {"Channel #"=9, "TC TYPE"=10086, "Name"=""}, {"Channel #"=13, "TC TYPE"=10086, "Name"=""}], "Channel Setup 3"=[{"Channel #"=1, "TC TYPE"=10086, "Name"=""}, {"Channel #"=5, "TC TYPE"=10086, "Name"=""}, {"Channel #"=9, "TC TYPE"=10086, "Name"=""}, {"Channel #"=13, "TC TYPE"=10086, "Name"=""}], "Channel Setup 4"=[{"Channel #"=1, "TC TYPE"=10086, "Name"=""}, {"Channel #"=5, "TC TYPE"=10086, "Name"=""}, {"Channel #"=9, "TC TYPE"=10086, "Name"=""}, {"Channel #"=13, "TC TYPE"=10086, "Name"=""}]} {"Channel Setup 4"."TC TYPE" items=["J"=10072, "K"=10073, "N"=10077, "R"=10082, "S"=10085, "T"=10086, "B"=10047, "E"=10055]; "Channel Setup 4"."Channel #" min=1 max=16 step=1; "Channel Setup 3"."TC TYPE" items=["J"=10072, "K"=10073, "N"=10077, "R"=10082, "S"=10085, "T"=10086, "B"=10047, "E"=10055]; "Channel Setup 3"."Channel #" min=1 max=16 step=1; "Channel Setup 2"."TC TYPE" items=["J"=10072, "K"=10073, "N"=10077, "R"=10082, "S"=10085, "T"=10086, "B"=10047, "E"=10055]; "Channel Setup 2"."Channel #" min=1 max=16 step=1; "Channel Setup"."TC TYPE" items=["J"=10072, "K"=10073, "N"=10077, "R"=10082, "S"=10085, "T"=10086, "B"=10047, "E"=10055]; "Channel Setup"."Channel #" min=1 max=16 step=1}
  out "IP Address 10":string=" "
  in  "Minutes between emails 10":dbl=10.0
  in  "Popout to new window 5":bool
  in  "Tab Control 6":T2
  in  "String 73":string
  out "DisplayCluster 5":T3={"Thermometer 2"=0.0, "Temperature Chart 4"=[{"t0"=timestamp(3419368924.4957023 s since 1904-01-01), "dt"=1.0, "Y"=[23.012484100583272], "attributes"=variant("NI_ChannelName"=variant(string "ai0"), "NI_UnitDescription"=variant(string "Deg C"))}, {"t0"=timestamp(3419368924.4957023 s since 1904-01-01), "dt"=1.0, "Y"=[23.20749068697193], "attributes"=variant("NI_ChannelName"=variant(string "ai1"), "NI_UnitDescription"=variant(string "Deg C"))}, {"t0"=timestamp(3419368924.4957023 s since 1904-01-01), "dt"=1.0, "Y"=[23.4994745351067], "attributes"=variant("NI_ChannelName"=variant(string "ai2"), "NI_UnitDescription"=variant(string "Deg C"))}], "Alarm"=FALSE, "Thermometer"=0.0, "File Path"=""} {"Thermometer" scale=0.0..100.0; "Thermometer 2" scale=0.0..100.0}
  out "Temperatures 5":dbl[](array[numeric]) format="%#.2f"
  in  "Reset max/min 5":bool
  in  "Save Data 5":bool=TRUE
  in  "Log File Path 5":path=path "c:/Temp/Data"
  out "DAQmx Device Name 5":tag="cDAQ2Mod1"
  out "Errors 5":errorcluster
  in  "Number of channels 5":i32=1 min=1 max=16 step=1
  in  "sample/S 5":dbl=1.0 min=0.1 max=75.0 step=0.1
  in  "Alarm recipients 5":string[](array[string])=["dconnors@intven.com"]
  in  "Upper Alarm 5":dbl=150.0
  in  "Lower Alarm 5":dbl=-150.0
  in  "Email Enable 5":bool
  in  "Cluster 6":T4={"Channel Setup"=[{"Channel #"=1, "TC TYPE"=10086, "Name"=""}, {"Channel #"=5, "TC TYPE"=10086, "Name"=""}, {"Channel #"=9, "TC TYPE"=10086, "Name"=""}, {"Channel #"=13, "TC TYPE"=10086, "Name"=""}], "Channel Setup 2"=[{"Channel #"=1, "TC TYPE"=10086, "Name"=""}, {"Channel #"=5, "TC TYPE"=10086, "Name"=""}, {"Channel #"=9, "TC TYPE"=10086, "Name"=""}, {"Channel #"=13, "TC TYPE"=10086, "Name"=""}], "Channel Setup 3"=[{"Channel #"=1, "TC TYPE"=10086, "Name"=""}, {"Channel #"=5, "TC TYPE"=10086, "Name"=""}, {"Channel #"=9, "TC TYPE"=10086, "Name"=""}, {"Channel #"=13, "TC TYPE"=10086, "Name"=""}], "Channel Setup 4"=[{"Channel #"=1, "TC TYPE"=10086, "Name"=""}, {"Channel #"=5, "TC TYPE"=10086, "Name"=""}, {"Channel #"=9, "TC TYPE"=10086, "Name"=""}, {"Channel #"=13, "TC TYPE"=10086, "Name"=""}]} {"Channel Setup 4"."TC TYPE" items=["J"=10072, "K"=10073, "N"=10077, "R"=10082, "S"=10085, "T"=10086, "B"=10047, "E"=10055]; "Channel Setup 4"."Channel #" min=1 max=16 step=1; "Channel Setup 3"."TC TYPE" items=["J"=10072, "K"=10073, "N"=10077, "R"=10082, "S"=10085, "T"=10086, "B"=10047, "E"=10055]; "Channel Setup 3"."Channel #" min=1 max=16 step=1; "Channel Setup 2"."TC TYPE" items=["J"=10072, "K"=10073, "N"=10077, "R"=10082, "S"=10085, "T"=10086, "B"=10047, "E"=10055]; "Channel Setup 2"."Channel #" min=1 max=16 step=1; "Channel Setup"."TC TYPE" items=["J"=10072, "K"=10073, "N"=10077, "R"=10082, "S"=10085, "T"=10086, "B"=10047, "E"=10055]; "Channel Setup"."Channel #" min=1 max=16 step=1}
  out "IP Address 5":string=" "
  in  "Minutes between emails 5":dbl=10.0
  in  "Minutes displayed 2":dbl=60.0
  in  "stop 2":bool
  out "Sensor 3 Temperature 2":waveform(dbl)(graph)={"t0"=timestamp(3552338969.221673 s since 1904-01-01), "dt"=0.001, "Y"=[19.008294294897723], "attributes"=variant("NI_ChannelName"=variant(string "Temp3"), "NI_UnitDescription"=variant(string "Amps"))}
  out "Sensor 3 Humidity 2":waveform(dbl)(graph)={"t0"=timestamp(3552338969.221658 s since 1904-01-01), "dt"=0.001, "Y"=[61.16415083954544], "attributes"=variant("NI_ChannelName"=variant(string "Humidity3"), "NI_UnitDescription"=variant(string "Amps"))}
  out "Sensor 2 Temperature 2":waveform(dbl)(graph)={"t0"=timestamp(3552338969.221643 s since 1904-01-01), "dt"=0.001, "Y"=[17.601047768518942], "attributes"=variant("NI_ChannelName"=variant(string "Temp2"), "NI_UnitDescription"=variant(string "Amps"))}
  out "Sensor 2 Humidity 2":waveform(dbl)(graph)={"t0"=timestamp(3552338969.221613 s since 1904-01-01), "dt"=0.001, "Y"=[70.37875059333966], "attributes"=variant("NI_ChannelName"=variant(string "Humidity2"), "NI_UnitDescription"=variant(string "Amps"))}
  out "Sensor 1 Temperature 2":waveform(dbl)(graph)={"t0"=timestamp(3552338969.221628 s since 1904-01-01), "dt"=0.001, "Y"=[17.486537818762628], "attributes"=variant("NI_ChannelName"=variant(string "Temp1"), "NI_UnitDescription"=variant(string "Amps"))}
  out "Sensor 1 Humidity 2":waveform(dbl)(graph)={"t0"=timestamp(3552338969.221598 s since 1904-01-01), "dt"=0.001, "Y"=[66.037122005], "attributes"=variant("NI_ChannelName"=variant(string "Humidity1"), "NI_UnitDescription"=variant(string "Amps"))}
  in  "Minutes displayed":dbl=60.0
  in  "stop":bool
  out "Sensor 3 Temperature":waveform(dbl)(graph)={"t0"=timestamp(3552338969.221673 s since 1904-01-01), "dt"=0.001, "Y"=[19.008294294897723], "attributes"=variant("NI_ChannelName"=variant(string "Temp3"), "NI_UnitDescription"=variant(string "Amps"))}
  out "Sensor 3 Humidity":waveform(dbl)(graph)={"t0"=timestamp(3552338969.221658 s since 1904-01-01), "dt"=0.001, "Y"=[61.16415083954544], "attributes"=variant("NI_ChannelName"=variant(string "Humidity3"), "NI_UnitDescription"=variant(string "Amps"))}
  out "Sensor 2 Temperature":waveform(dbl)(graph)={"t0"=timestamp(3552338969.221643 s since 1904-01-01), "dt"=0.001, "Y"=[17.601047768518942], "attributes"=variant("NI_ChannelName"=variant(string "Temp2"), "NI_UnitDescription"=variant(string "Amps"))}
  out "Sensor 2 Humidity":waveform(dbl)(graph)={"t0"=timestamp(3552338969.221613 s since 1904-01-01), "dt"=0.001, "Y"=[70.37875059333966], "attributes"=variant("NI_ChannelName"=variant(string "Humidity2"), "NI_UnitDescription"=variant(string "Amps"))}
  out "Sensor 1 Temperature":waveform(dbl)(graph)={"t0"=timestamp(3552338969.221628 s since 1904-01-01), "dt"=0.001, "Y"=[17.486537818762628], "attributes"=variant("NI_ChannelName"=variant(string "Temp1"), "NI_UnitDescription"=variant(string "Amps"))}
  out "Sensor 1 Humidity":waveform(dbl)(graph)={"t0"=timestamp(3552338969.221598 s since 1904-01-01), "dt"=0.001, "Y"=[66.037122005], "attributes"=variant("NI_ChannelName"=variant(string "Humidity1"), "NI_UnitDescription"=variant(string "Amps"))}
  out "Waveform Chart 2":dbl(graph)
  out "Waveform Chart":dbl(graph)
  in  "Analog out 17":dbl
  in  "Analog out 4":dbl
  in  "Analog out 3":dbl
  in  "Analog out 16":dbl
  in  "Analog out 2":dbl
  in  "Analog out 1":dbl
  in  "Value 20":string
  in  "THEN 10":u16(ring) items=["Relay 1", "TC mod 1 ch 1"]
  in  "Value 19":string
  in  "Condition 10":u16(ring) items=["!=", "==", "<=", ">=", "<", ">"]
  in  "IF 10":u16(ring) items=["TC mod 1 ch 1"]
  in  "Value 18":string
  in  "THEN 9":u16(ring) items=["Relay 1", "TC mod 1 ch 1"]
  in  "Value 17":string
  in  "Condition 9":u16(ring) items=["!=", "==", "<=", ">=", "<", ">"]
  in  "IF 9":u16(ring) items=["TC mod 1 ch 1"]
  in  "Value 16":string
  in  "THEN 8":u16(ring) items=["Relay 1", "TC mod 1 ch 1"]
  in  "Value 15":string
  in  "Condition 8":u16(ring) items=["!=", "==", "<=", ">=", "<", ">"]
  in  "IF 8":u16(ring) items=["TC mod 1 ch 1"]
  in  "Value 14":string
  in  "THEN 7":u16(ring) items=["Relay 1", "TC mod 1 ch 1"]
  in  "Value 13":string
  in  "Condition 7":u16(ring) items=["!=", "==", "<=", ">=", "<", ">"]
  in  "IF 7":u16(ring) items=["TC mod 1 ch 1"]
  in  "Value 12":string
  in  "THEN 6":u16(ring) items=["Relay 1", "TC mod 1 ch 1"]
  in  "Value 11":string
  in  "Condition 6":u16(ring) items=["!=", "==", "<=", ">=", "<", ">"]
  in  "IF 6":u16(ring) items=["TC mod 1 ch 1"]
  in  "Value 10":string
  in  "THEN 5":u16(ring) items=["Relay 1", "TC mod 1 ch 1"]
  in  "Value 9":string
  in  "Condition 5":u16(ring) items=["!=", "==", "<=", ">=", "<", ">"]
  in  "IF 5":u16(ring) items=["TC mod 1 ch 1"]
  in  "Value 8":string
  in  "THEN 4":u16(ring) items=["Relay 1", "TC mod 1 ch 1"]
  in  "Value 7":string
  in  "Condition 4":u16(ring) items=["!=", "==", "<=", ">=", "<", ">"]
  in  "IF 4":u16(ring) items=["TC mod 1 ch 1"]
  in  "Value 6":string
  in  "THEN 3":u16(ring) items=["Relay 1", "TC mod 1 ch 1"]
  in  "Value 5":string
  in  "Condition 3":u16(ring) items=["!=", "==", "<=", ">=", "<", ">"]
  in  "IF 3":u16(ring) items=["TC mod 1 ch 1"]
  in  "Value 3":string
  in  "THEN 2":u16(ring) items=["Relay 1", "TC mod 1 ch 1"]
  in  "Value 2":string
  in  "Condition 2":u16(ring) items=["!=", "==", "<=", ">=", "<", ">"]
  in  "IF 2":u16(ring) items=["TC mod 1 ch 1"]
  in  "Value 4":string
  in  "THEN":u16(ring) items=["Relay 1", "TC mod 1 ch 1"]
  in  "Value":string
  in  "Condition":u16(ring) items=["!=", "==", "<=", ">=", "<", ">"]
  in  "IF":u16(ring) items=["TC mod 1 ch 1"]
  in  "OK Button 2":bool
  in  "Loop profile at end 2":bool
  out "Profile started 2":timestamp
  out "Profile loaded 2":string
  in  "Time Stamp 2":timestamp
  in  "Start profile at time 2":bool
  in  "Start profile now 2":bool
  out "Loaded profiles 2":dbl(graph)
  in  "Load profile 2":path
  in  "OK Button":bool
  in  "Loop profile at end":bool
  out "Profile started":timestamp
  out "Profile loaded":string
  in  "Time Stamp":timestamp
  in  "Start profile at time":bool
  in  "Start profile now":bool
  out "Loaded profiles":dbl(graph)
  in  "Load profile":path
  in  "Control 6":enum32{"Radio Selection 1", "Radio Selection 2"}(radio)
  in  "Freq 4":dbl
  in  "Current limit 6":dbl
  in  "Volts 6":dbl
  in  "Freq 3":dbl
  in  "Control 5":enum32{"Radio Selection 1", "Radio Selection 2"}(radio)
  in  "Current limit 5":dbl
  in  "Volts 5":dbl
  in  "Control 4":enum32{"Radio Selection 1", "Radio Selection 2"}(radio)
  in  "Current limit 4":dbl
  in  "Volts 4":dbl
  out "DC source 2":dbl(graph)
  out "AC source 4":dbl(graph)
  out "AC source 3":dbl(graph)
  in  "Control 3":enum32{"Radio Selection 1", "Radio Selection 2"}(radio)
  in  "Freq 2":dbl
  in  "Current limit 3":dbl
  in  "Volts 3":dbl
  in  "Freq":dbl
  in  "Control 2":enum32{"Radio Selection 1", "Radio Selection 2"}(radio)
  in  "Current limit 2":dbl
  in  "Volts 2":dbl
  in  "Control":enum32{"Radio Selection 1", "Radio Selection 2"}(radio)
  in  "Current limit":dbl
  in  "Volts":dbl
  out "DC source":dbl(graph)
  out "AC source 2":dbl(graph)
  out "AC source 1":dbl(graph)
  # "Temperature"
  # "Humidity"
  # "Notes:\n1.  All names muse be unique\n2.  Sample/S range 0.1 to 75\n3."
  # "Only Works when on intven.com"
  # "May take upto 10sec to take effect"
  # "Notes:\n1.  All names muse be unique\n2.  Sample/S range 0.1 to 75\n3."
  # "Only Works when on intven.com"
  # "Notes:\n1.  All names muse be unique\n2.  Sample/S range 0.1 to 75\n3."
  # "Only Works when on intven.com"
  # "May take upto 10sec to take effect"
  # "Notes:\n1.  All names muse be unique\n2.  Sample/S range 0.1 to 75\n3."
  # "Only Works when on intven.com"
  # "Notes:\n1.  All names muse be unique\n2.  Sample/S range 0.1 to 75\n3."
  # "Only Works when on intven.com"
  # "May take upto 10sec to take effect"
  # "Notes:\n1.  All names muse be unique\n2.  Sample/S range 0.1 to 75\n3."
  # "Only Works when on intven.com"
  # "Notes:\n1.  All names muse be unique\n2.  Sample/S range 0.1 to 75\n3."
  # "Only Works when on intven.com"
  # "May take upto 10sec to take effect"
  # "Notes:\n1.  All names muse be unique\n2.  Sample/S range 0.1 to 75\n3."
  # "Only Works when on intven.com"
  # "Notes:\n1.  All names muse be unique\n2.  Sample/S range 0.1 to 75\n3."
  # "Only Works when on intven.com"
  # "May take upto 10sec to take effect"
  # "Notes:\n1.  All names muse be unique\n2.  Sample/S range 0.1 to 75\n3."
  # "Only Works when on intven.com"
  # "Chamber Temperatures and Humidities as reported by Omega boxes on walls"
  # "Chamber Temperatures and Humidities as reported by Omega boxes on walls"
  # "="
  # "="
  # "="
  # "="
  # "="
  # "="
  # "="
  # "="
  # "="
  # "="
  # "if condition send alarm email"
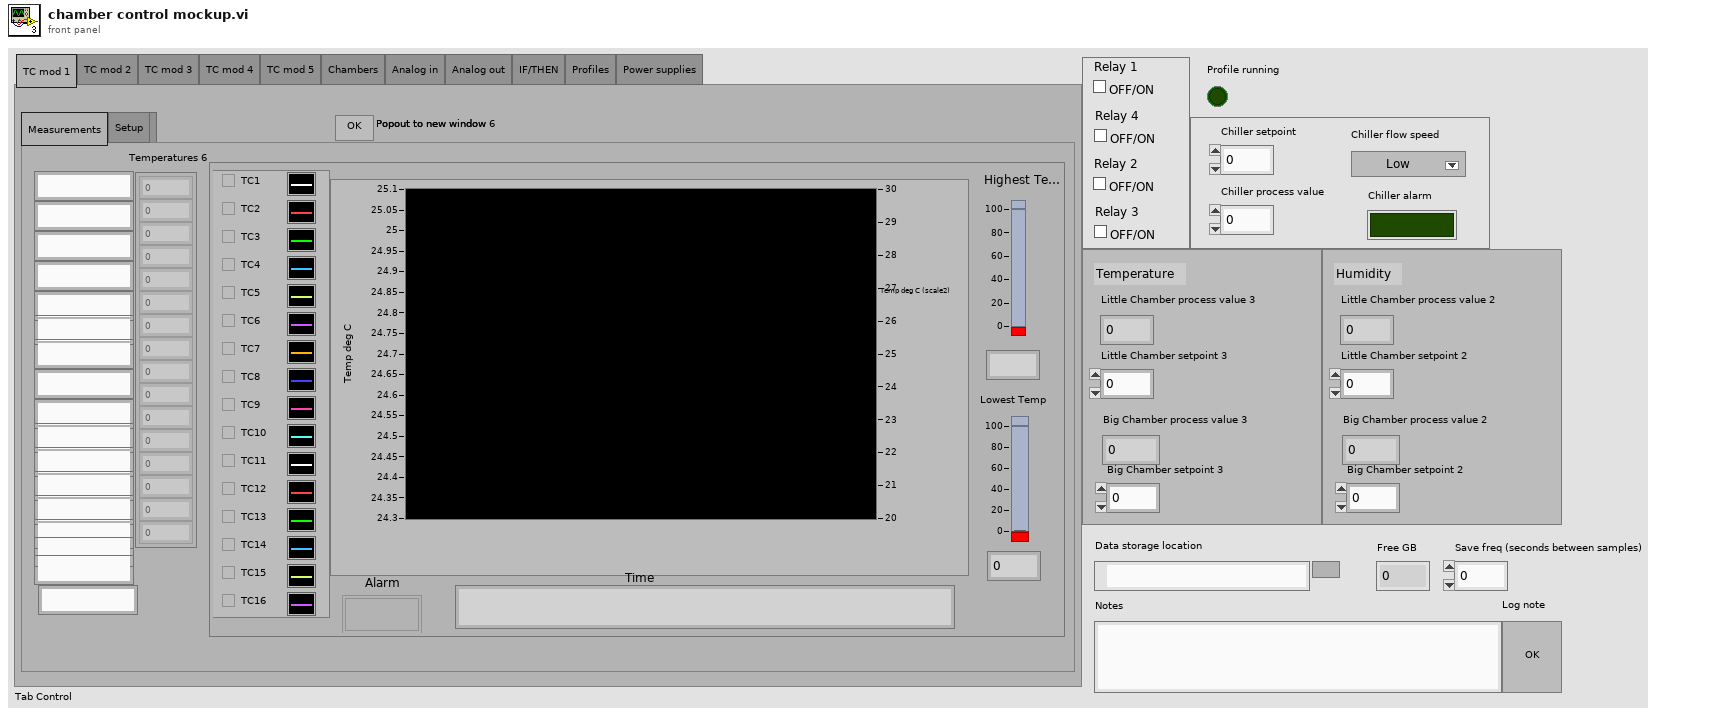
[diagram p1: front panel]
types:
  T1 = enum32{"TC mod 1", "TC mod 2", "TC mod 3", "TC mod 4", "TC mod 5", "Chambers", "Analog in", "Analog out", "IF/THEN", "Profiles", "Power supplies"}
  T2 = typedef "TabControl.ctl" = enum32{"Measurements", "Setup"}
  T3 = typedef "outputcluster.ctl" = cluster{"Thermometer 2":dbl, "Temperature Chart 4":waveform(dbl)[], "Alarm":bool, "Thermometer":dbl, "File Path":string}
  T4 = typedef "TemperatureControlCluster2.ctl" = cluster{"Channel Setup":cluster{"Channel #":i8, "TC TYPE":i32, "Name":string}[], "Channel Setup 2":cluster{"Channel #":i8, "TC TYPE":i32, "Name":string}[], "Channel Setup 3":cluster{"Channel #":i8, "TC TYPE":i32, "Name":string}[], "Channel Setup 4":cluster{"Channel #":i8, "TC TYPE":i32, "Name":string}[]}
diagram:
